vi "LeyboldTurbo_Main.vi"() -> ()   [LabVIEW 2019]
doc: "Example VI to demonstrate the use of the Oerlikon Leybold TMP driver."
uses:
  <instrlib>/Leybold TURBOVAC/Leybold TURBOVAC.lvlib
panel:
  in  "remote_cont_2":bool caption="Remote Control"
  in  "reconn":bool
  out "meter_freq":cluster{dbl, dbl}(knob) caption="Frequency (Hz)" scale=0.0..700.0 scale format="%#.2f"
  in  "Tab Control":T1(tab)
  out "status_word_1":T2 caption="Status words 1"
  out "status_word_2":T2 caption="Status words 2"
  out "chart_freq":waveform(dbl)[](graph)
  out "chart_curr":waveform(dbl)[](graph)
  out "chart_temp":waveform(dbl)[](graph)
  in  "VISA2":refnum<visa-resource-name>="COM43"
  in  "VISA1":refnum<visa-resource-name>="COM44" caption="VISA"
  out "status_comm_2":bool caption="Comm. status"
  in  "operate_2":bool caption="Operate"
  out "temp_2":i32 caption="Temperature"
  out "current_2":dbl format="%.1f"
  out "freq_2":u16
  out "current_1":dbl caption="Current" format="%.1g"
  out "freq_1":u16 caption="Frequency"
  in  "SN":string[](array[string])=["240804202", "240804204"]
  out "temp_1":i32 caption="Temperature"
  out "time_meas":timestamp caption="Last update" format="%<%Y-%m-%d %H:%M:%S>T"
  out "status_comm_1":bool caption="Comm. status"
  in  "interval":u32=1000 caption="Interval"
  in  "remote_cont_1":bool caption="Remote \nControl"
  in  "operate_1":bool caption="Operate"
  in  "stop":bool
  # "IVC Turbo Pumps"
  # "Leybold TURBOVAC 1350iR + TURBO.DRIVE 500e"
  # "Turbo #1"
  # "Turbo #2"
  # "ms"
  # "Turbo #1"
  # "Turbo #2"
  # "Hz"
  # "Hz"
  # "A"
  # "A"
  # "°C"
  # "°C"
  # "Turbo #1\nTurbo #2"
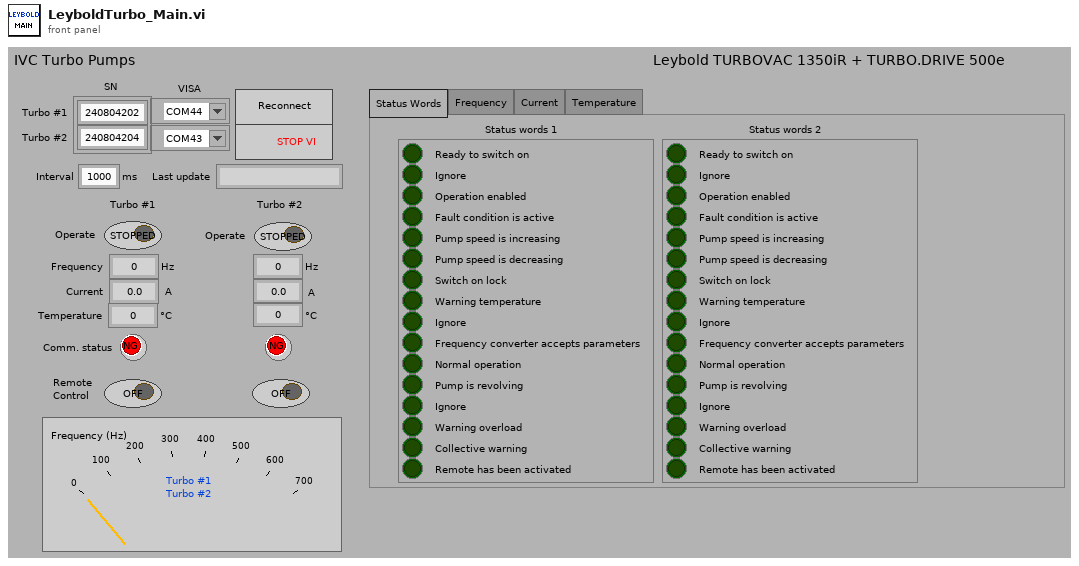
[diagram p1: front panel]
types:
  T1 = enum32{"Status Words", "Frequency", "Current", "Temperature"}
  T2 = cluster{"Ready to switch on":bool, "Ignore":bool, "Operation enabled":bool, "Fault condition is active":bool, "Pump speed is increasing":bool, "Pump speed is decreasing":bool, "Switch on lock":bool, "Warning temperature":bool, "Ignore":bool, "Frequency converter accepts parameters":bool, "Normal operation":bool, "Pump is revolving":bool, "Ignore":bool, "Warning overload":bool, "Collective warning":bool, "Remote has been activated":bool}
  T3 = typedef "Leybold TURBOVAC.lvlib/Device Parameters Indicator.ctl" = cluster{"Length of data block":u8, "Converter address":u8, "Converter type":T4, "PZD1":u16, "PZD2":u16}
  T4 = typedef "Leybold TURBOVAC.lvlib/Converter Type Indicator.ctl" = u16
  T5 = enum8{"Enabled", "Disabled", "Disabled and Grayed Out"}
  T6 = cluster{"Actual stator frequency [Hz]":u16, "Converter temperature [°C]":u16, "Motor current [A]":dbl, "Intermediate circuit voltage Uzk [V]":dbl}
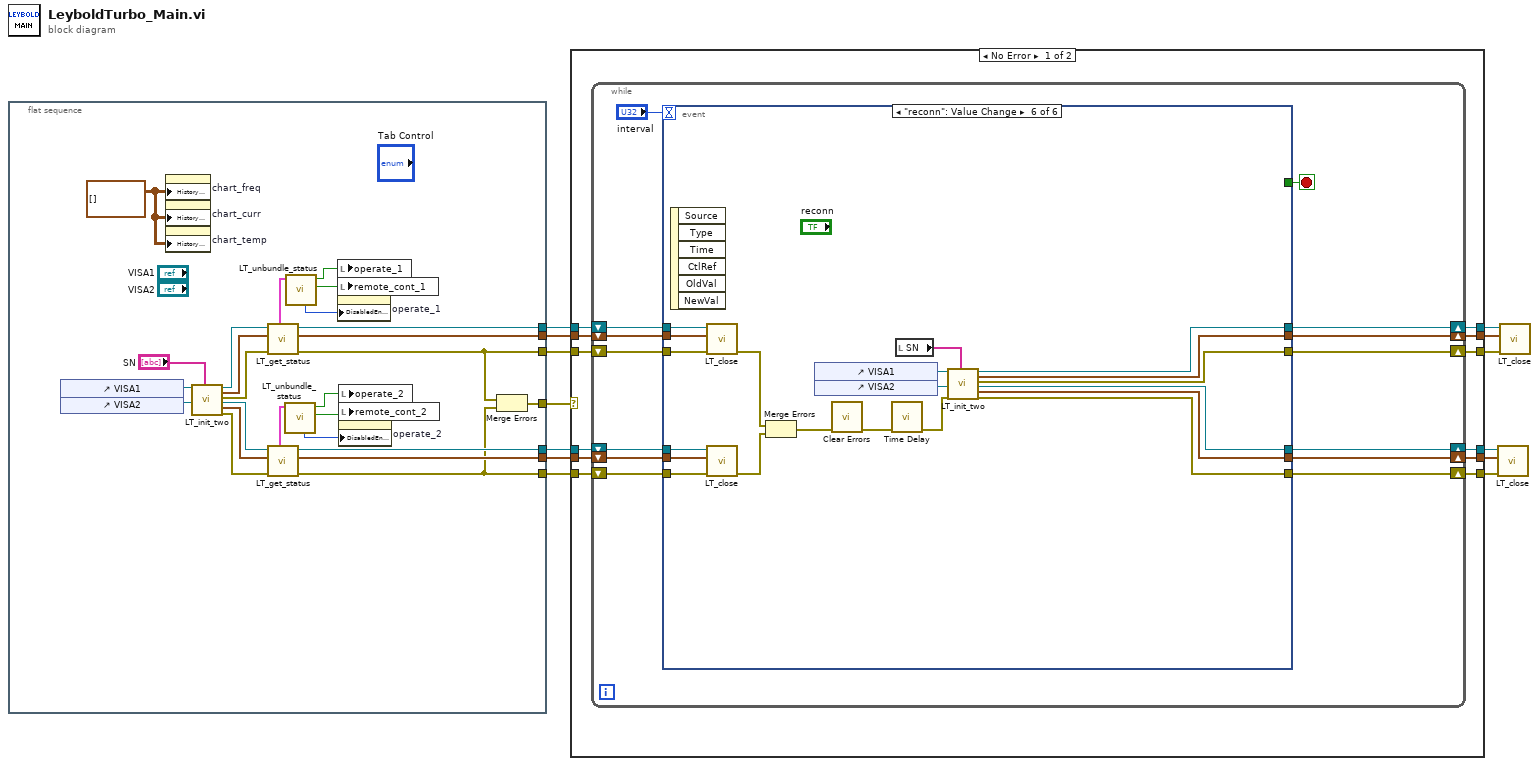
[diagram p0: block diagram]
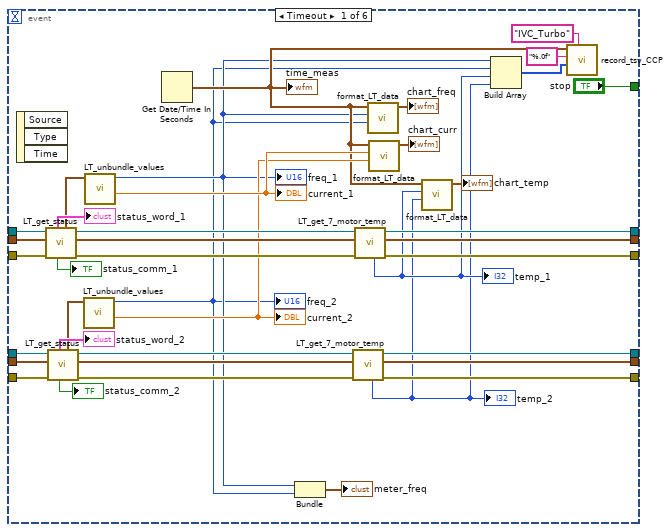
[diagram p2: hidden frame]
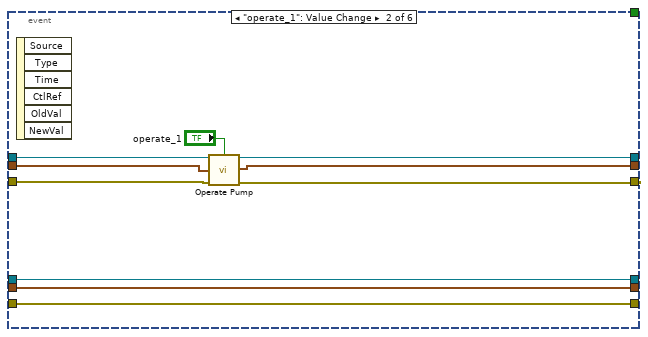
[diagram p3: hidden frame]
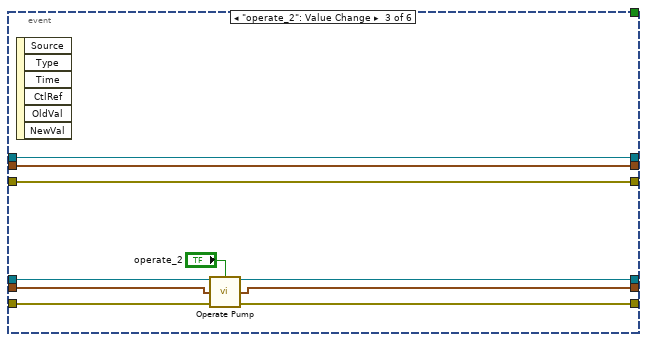
[diagram p4: hidden frame]
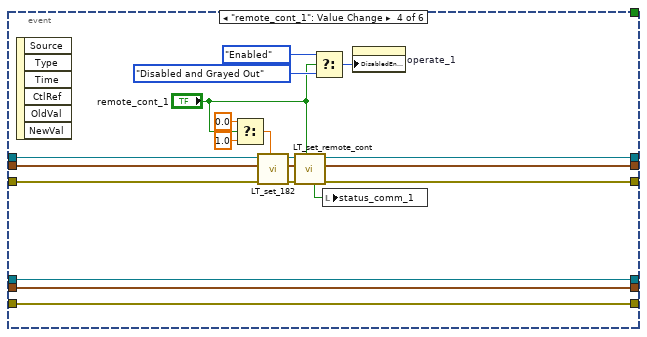
[diagram p5: hidden frame]
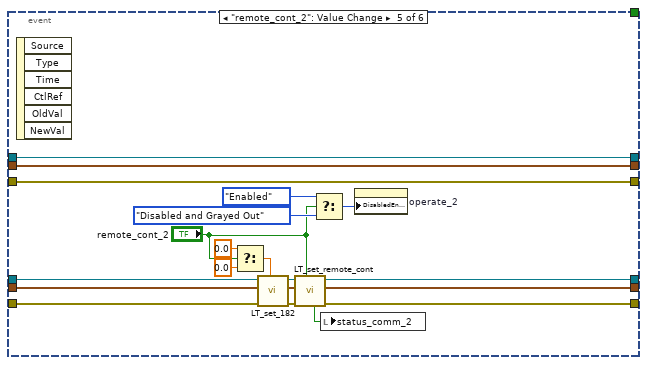
[diagram p6: hidden frame]
diagram:
  n1 = flat-sequence {
    tunnel: [w31] -> w10
    tunnel: [w32] -> w9
    tunnel: [w25] -> w8
    tunnel: [w24] -> w7
    tunnel: [w28] -> w6
    tunnel: [w23] -> w5
    tunnel: [w38] -> w4
    frame #0 {
      w37 = waveform(dbl)[][] [] ("History Data")
      n2 = control-ref of="VISA1"() -> (w36:refnum<vi>)
      n3 = control-ref of="VISA2"() -> (w35:refnum<vi>)
      n4 = property on="chart_freq" class="WFChart (strict)"("History Data"=w37) -> ()  [unwired: 2 in, 2 out]
      n5 = property on="chart_curr" class="WFChart (strict)"("History Data"=w37) -> ()  [unwired: 2 in, 2 out]
      n6 = property on="chart_temp" class="WFChart (strict)"("History Data"=w37) -> ()  [unwired: 2 in, 2 out]
      n7 = call "LT_init_two.vi"("VISA1"=w36, "VISA2"=w35, "SN"="SN") -> ("VISA1 out"=w33:refnum<visa-resource-name>, "dev_param_1"=w30:T3, "error1"=w29:errorcluster, "VISA2 out"=w26:refnum<visa-resource-name>, "dev_param_2"=w21:T3, "error2"=w22:errorcluster)  [unwired: 11 in]
      n8 = call "LT_get_status.vi"("error in"=w29, "dev_param_in"=w30, "VISA in"=w33) -> ("error out"=w28:errorcluster, "dev_param_out"=w31:T3, "VISA out"=w32:refnum<visa-resource-name>, "Status word"=w27:T2)  [unwired: 1 in, 4 out]
      n9 = call "LT_get_status.vi"("error in"=w22, "dev_param_in"=w21, "VISA in"=w26) -> ("error out"=w23:errorcluster, "dev_param_out"=w24:T3, "VISA out"=w25:refnum<visa-resource-name>, "Status word"=w20:T2)  [unwired: 1 in, 4 out]
      n10 = call "LT_unbundle_status.vi"("Status word"=w20) -> ("Remote has been activated"=w19:bool, "Operation enabled"=w14:bool, "enabled"=w17:T5)  [unwired: 8 in]
      n11 = call "LT_unbundle_status.vi"("Status word"=w27) -> ("Remote has been activated"=w15:bool, "Operation enabled"=w16:bool, "enabled"=w18:T5)  [unwired: 8 in]
      n12 = local write "operate_1"(w16) -> ()
      n13 = local write "remote_cont_1"(w15) -> ()
      n14 = property on="operate_1" class="Bool (strict)"("DisabledEnum"=w18) -> ()  [unwired: 2 in, 2 out]
      n15 = local write "operate_2"(w14) -> ()
      n16 = local write "remote_cont_2"(w19) -> ()
      n17 = property on="operate_2" class="Bool (strict)"("DisabledEnum"=w17) -> ()  [unwired: 2 in, 2 out]
      n18 = Merge Errors(w28, w23) -> (w38:errorcluster)
    }
  }
  n19 = case shown="No Error" w4 {
    tunnel: w9 -> [w47 w188]
    tunnel: w10 -> [w40 w189]
    tunnel: [w50 w188] -> w13
    tunnel: [w49 w189] -> w11
    tunnel: [w48 w187] -> w12
    tunnel: w8 -> [w45 w186]
    tunnel: w7 -> [w39 w184]
    tunnel: w5 -> [w44 w185]
    tunnel: w6 -> [w46 w187]
    tunnel: [w43 w186] -> w3
    tunnel: [w41 w185] -> w2
    tunnel: [w42 w184] -> w1
    frame No Error {
      n20 = while {
        shift-right: [w59] -> w49
        shift-left: w40 -> [w60]
        shift-right: [w58] -> w48
        shift-left: w46 -> [w62]
        shift-right: [w63] -> w50
        shift-left: w47 -> [w61]
        shift-right: [w53] -> w43
        shift-left: w45 -> [w56]
        shift-right: [w52] -> w42
        shift-left: w39 -> [w54]
        shift-right: [w51] -> w41
        shift-left: w44 -> [w55]
        stop <- w64 stop-if-true
        n21 = event shown="[5] \"reconn\": Value Change" {
          selector: _ -> [_ _ _ _ _ _]
          dyn-events: _ -> [_ _ _ _ _ _]
          timeout: "interval" -> [_ _ _ _ _ _]
          tunnel: ["stop" _ _ _ _ _] -> w64
          tunnel: [w96 w109 w116 w142 w151 w183] -> w63
          tunnel: w62 -> [w101 w110 w114 w129 w150 w172]
          tunnel: w61 -> [w102 w112 w116 w133 w151 w174]
          tunnel: w60 -> [w100 w111 w115 w128 w149 w173]
          tunnel: [w94 w108 w115 w141 w149 w182] -> w59
          tunnel: [w92 w107 w114 w143 w150 w181] -> w58
          tunnel: w56 -> [w91 w106 w122 w140 w153 w171]
          tunnel: w55 -> [w90 w104 w121 w139 w148 w170]
          tunnel: w54 -> [w89 w105 w120 w134 w146 w169]
          tunnel: [w85 w106 w119 w140 w152 w180] -> w53
          tunnel: [w84 w105 w117 w134 w145 w179] -> w52
          tunnel: [w83 w104 w118 w139 w147 w178] -> w51
          event Timeout {
            n22 = event-data() -> ()  [unwired: 1 in, 3 out]
            n23 = call "LT_get_status.vi"("error in"=w101, "dev_param_in"=w100, "VISA in"=w102) -> ("error out"=w93:errorcluster, "dev_param_out"=w95:T3, "VISA out"=w97:refnum<visa-resource-name>, "Status values"=w82:T6, "status_comm"=→"status_comm_1":bool, "Status word"=→"status_word_1":T2)  [unwired: 1 in, 2 out]
            n24 = call "LT_get_status.vi"("error in"=w90, "dev_param_in"=w89, "VISA in"=w91) -> ("error out"=w87:errorcluster, "dev_param_out"=w86:T3, "VISA out"=w88:refnum<visa-resource-name>, "Status values"=w74:T6, "status_comm"=→"status_comm_2":bool, "Status word"=→"status_word_2":T2)  [unwired: 1 in, 2 out]
            n25 = call "LT_unbundle_values.vi"("Status values"=w74) -> ("current"=w73:dbl, "freq"=w69:u16)  [unwired: 7 in, 2 out]
            "freq_2" <- w69
            "current_2" <- w73
            n26 = call "LT_unbundle_values.vi"("Status values"=w82) -> ("current"=w75:dbl, "freq"=w70:u16)  [unwired: 7 in, 2 out]
            "freq_1" <- w70
            "current_1" <- w75
            n27 = Get Date/Time In Seconds() -> (seconds since 1Jan1904=w72:timestamp)
            "time_meas" <- w72
            n28 = Bundle("freq"=w70, "freq"=w69) -> (→"meter_freq":cluster{"freq":u16, "freq":u16})  [unwired: 1 in]
            n29 = call "LT_get_7_motor_temp.vi"("error in"=w87, "dev_param_in"=w86, "VISA in"=w88) -> ("error out"=w83:errorcluster, "dev_param_out"=w84:T3, "VISA out"=w85:refnum<visa-resource-name>, "temp"=w67:i32)  [unwired: 5 in]
            "temp_2" <- w67
            n30 = call "LT_get_7_motor_temp.vi"("error in"=w93, "dev_param_in"=w95, "VISA in"=w97) -> ("error out"=w92:errorcluster, "dev_param_out"=w94:T3, "VISA out"=w96:refnum<visa-resource-name>, "temp"=w68:i32)  [unwired: 5 in]
            "temp_1" <- w68
            n31 = call "format_LT_data.vi"("value_2"=w69, "value_1"=w70, "time"=w72) -> ("waveform_array"=→"chart_freq":waveform(dbl)[])  [unwired: 8 in]
            n32 = call "format_LT_data.vi"("value_2"=w73, "value_1"=w75, "time"=w72) -> ("waveform_array"=→"chart_curr":waveform(dbl)[])  [unwired: 8 in]
            n33 = call "format_LT_data.vi"("value_2"=w67, "value_1"=w68, "time"=w72) -> ("waveform_array"=→"chart_temp":waveform(dbl)[])  [unwired: 8 in]
            n34 = Build Array(w70, w69, w68, w67) -> (w71:i32[])
            n35 = call "record_tsv_CCP.vi"("folder_name"="IVC_Turbo", "value_array"=w71, "format"="%.0f", "time"=w72) -> ()  [unwired: 6 in, 2 out]
          }
          event "operate_1": Value Change {
            n36 = event-data() -> ()  [unwired: 1 in, 6 out]
            n37 = call <instrlib>:"Operate Pump.vi"("VISA resource name"=w112, "Operate pump (F: off)"="operate_1", "Device parameters"=w111, "error in (no error)"=w110) -> ("VISA resource name out"=w109:refnum<visa-resource-name>, "Device parameters out"=w108:T3, "error out"=w107:errorcluster)  [unwired: 9 in]
          }
          event "operate_2": Value Change {
            n38 = event-data() -> ()  [unwired: 1 in, 6 out]
            n39 = call <instrlib>:"Operate Pump.vi"("VISA resource name"=w122, "Operate pump (F: off)"="operate_2", "Device parameters"=w120, "error in (no error)"=w121) -> ("VISA resource name out"=w119:refnum<visa-resource-name>, "Device parameters out"=w117:T3, "error out"=w118:errorcluster)  [unwired: 9 in]
          }
          event "remote_cont_1": Value Change {
            n40 = event-data() -> ()  [unwired: 1 in, 6 out]
            n41 = Select(t=0.0, s="remote_cont_1", f=1.0) -> (s? t:f=w126:dbl)
            n42 = call "LT_set_182.vi"("sec"=w126, "error in"=w129, "dev_param_in"=w128, "VISA in"=w133) -> ("error out"=w130:errorcluster, "dev_param_out"=w131:T3, "VISA out"=w132:refnum<visa-resource-name>)  [unwired: 4 in, 1 out]
            n43 = call "LT_set_remote_cont.vi"("remote_cont"="remote_cont_1", "error in"=w130, "dev_param_in"=w131, "VISA in"=w132) -> ("error out"=w143:errorcluster, "dev_param_out"=w141:T3, "VISA out"=w142:refnum<visa-resource-name>, "status"=w138:bool)  [unwired: 4 in]
            n44 = Select(t=T5."Enabled" ("Disabled"), s="remote_cont_1", f=T5."Disabled and Grayed Out" ("Disabled")) -> (s? t:f=w137:T5)
            n45 = local write "status_comm_1"(w138) -> ()
            n46 = property on="operate_1" class="Bool (strict)"("DisabledEnum"=w137) -> ()  [unwired: 2 in, 2 out]
          }
          event "remote_cont_2": Value Change {
            n47 = event-data() -> ()  [unwired: 1 in, 6 out]
            n48 = Select(t=0.0, s="remote_cont_2", f=0.0) -> (s? t:f=w156:dbl)
            n49 = call "LT_set_182.vi"("sec"=w156, "error in"=w148, "dev_param_in"=w146, "VISA in"=w153) -> ("error out"=w158:errorcluster, "dev_param_out"=w159:T3, "VISA out"=w160:refnum<visa-resource-name>)  [unwired: 4 in, 1 out]
            n50 = call "LT_set_remote_cont.vi"("remote_cont"="remote_cont_2", "error in"=w158, "dev_param_in"=w159, "VISA in"=w160) -> ("error out"=w147:errorcluster, "dev_param_out"=w145:T3, "VISA out"=w152:refnum<visa-resource-name>, "status"=w144:bool)  [unwired: 4 in]
            n51 = Select(t=T5."Enabled" ("Disabled"), s="remote_cont_2", f=T5."Disabled and Grayed Out" ("Disabled")) -> (s? t:f=w163:T5)
            n52 = local write "status_comm_2"(w144) -> ()
            n53 = property on="operate_2" class="Bool (strict)"("DisabledEnum"=w163) -> ()  [unwired: 2 in, 2 out]
          }
          event "reconn": Value Change {
            n54 = event-data() -> ()  [unwired: 1 in, 6 out]
            n55 = call "LT_close.vi"("error in"=w172, "dev_param_in"=w173, "VISA in"=w174) -> ("error out"=w166:errorcluster)  [unwired: 8 in]
            n56 = call "LT_close.vi"("error in"=w170, "dev_param_in"=w169, "VISA in"=w171) -> ("error out"=w167:errorcluster)  [unwired: 8 in]
            n57 = Merge Errors(w166, w167) -> (w165:errorcluster)
            n58 = control-ref of="VISA1"() -> (w176:refnum<vi>)
            n59 = control-ref of="VISA2"() -> (w175:refnum<vi>)
            n60 = call <vilib>:"Clear Errors.vi"("error in (no error)"=w165) -> ("error out"=w164:errorcluster)  [unwired: 5 in, 1 out]
            n61 = call "Time Delay"("error in (no error)"=w164) -> ("error out"=w168:errorcluster)  [unwired: 10 in]
            n62 = local read "SN"() -> (w177:string[])
            n63 = call "LT_init_two.vi"("VISA1"=w176, "VISA2"=w175, "error in"=w168, "SN"=w177) -> ("VISA1 out"=w183:refnum<visa-resource-name>, "dev_param_1"=w182:T3, "error1"=w181:errorcluster, "VISA2 out"=w180:refnum<visa-resource-name>, "dev_param_2"=w179:T3, "error2"=w178:errorcluster)  [unwired: 10 in]
          }
        }
      }
    }
    frame Error {
    }
  }
  n64 = call "LT_close.vi"("error in"=w2, "dev_param_in"=w1, "VISA in"=w3) -> ()  [unwired: 8 in, 1 out]
  n65 = call "LT_close.vi"("error in"=w12, "dev_param_in"=w11, "VISA in"=w13) -> ()  [unwired: 8 in, 1 out]
